vi "Create Repeatability Results Summary Table.vi"(8 "error in (no error)":errorcluster, 11 "Repeatability Results":T1[](array[typedef]) {"Repeatability Percent FS" format="%#_3g"}) -> (0 "error out":errorcluster, 3 "Repeatability Table":string[][](array[string]))   [LabVIEW 2026, in "Analysis.lvlib"]
uses:
  Analysis.lvlib
  Repeatability Result.ctl
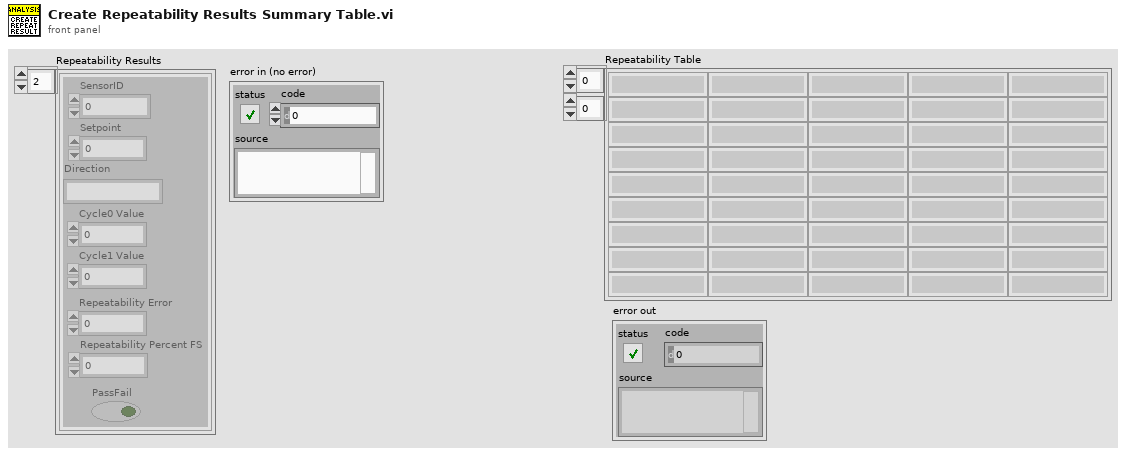
[diagram p1: front panel]
types:
  T1 = typedef "Analysis.lvlib/Repeatability Result.ctl" = cluster{"Setpoint":dbl, "Cycle0 Value":dbl, "SensorID":i32, "Cycle1 Value":dbl, "Repeatability Error":dbl, "Direction":string, "Repeatability Percent FS":dbl, "PassFail":bool}
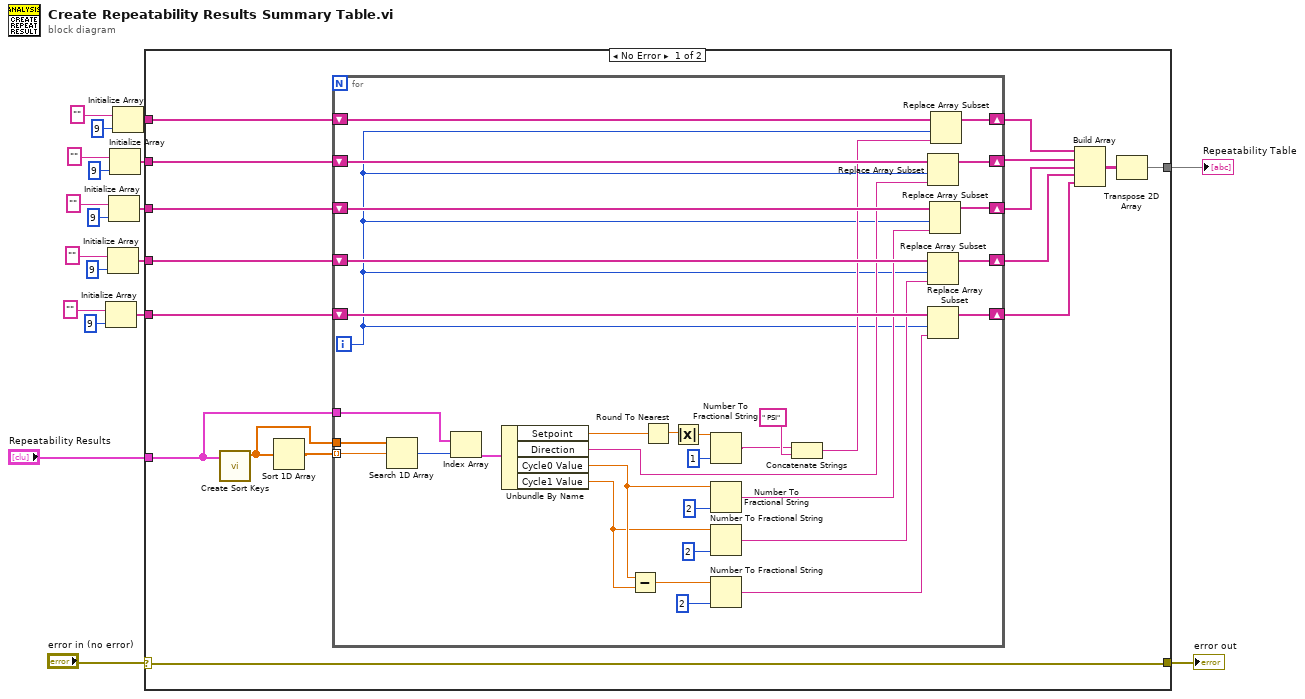
[diagram p0: block diagram]
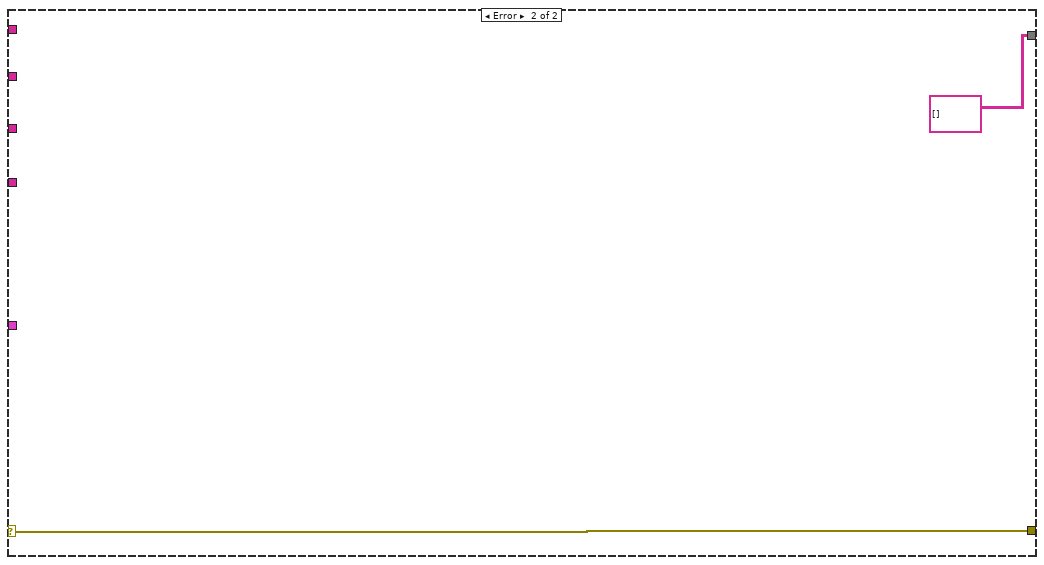
[diagram p2: hidden frame]
diagram:
  n1 = Initialize Array("" ("element"), 9 ("dimension size")) -> (w1:string[])
  n2 = Initialize Array("" ("element"), 9 ("dimension size")) -> (w4:string[])
  n3 = Initialize Array("" ("element"), 9 ("dimension size")) -> (w11:string[])
  n4 = Initialize Array("" ("element"), 9 ("dimension size")) -> (w14:string[])
  n5 = Initialize Array("" ("element"), 9 ("dimension size")) -> (w17:string[])
  n6 = case shown="No Error" "error in (no error)" {
    selector: "error in (no error)" -> [w27 w70]
    tunnel: w17 -> [w35 _]
    tunnel: w14 -> [w34 _]
    tunnel: w11 -> [w33 _]
    tunnel: "Repeatability Results" -> [w21 _]
    tunnel: [w28 string[][] []] -> w10
    tunnel: [w27 w70] -> w8
    tunnel: w4 -> [w26 _]
    tunnel: w1 -> [w24 _]
    frame No Error {
      n7 = call "Create Sort Keys.vi"("Repeatability Results"=w21) -> ("Sort Keys"=w20:dbl[])  [unwired: 9 in, 1 out]
      n8 = Sort 1D Array(array=w20) -> (sorted array=w22:dbl[])
      n9 = for {
        shift-right: [w65] -> w32
        shift-left: w35 -> [w68]
        shift-right: [w66] -> w31
        shift-left: w34 -> [w67]
        shift-right: [w63] -> w30
        shift-left: w33 -> [w64]
        shift-right: [w61] -> w25
        shift-left: w26 -> [w62]
        shift-right: [w59] -> w23
        shift-left: w24 -> [w60]
        tunnel: w22 -> [w52] mode=indexing
        tunnel: w20 -> [w51]
        tunnel: w21 -> [w49]
        i -> [w53]
        n10 = Search 1D Array(1D array=w51, element=w52) -> (index of element=w50:i32)  [unwired: 1 in]
        n11 = Index Array(array=w49, index=w50) -> (element=w36:T1)
        n12 = Unbundle By Name(w36) -> ("Setpoint"=w46:dbl, "Direction"=w57:string, "Cycle0 Value"=w40:dbl, "Cycle1 Value"=w39:dbl)
        n13 = Subtract(x=w40, y=w39) -> (x-y=w37:dbl)
        n14 = Round To Nearest(number=w46) -> (nearest integer value=w44:dbl)
        n15 = Absolute Value(x=w44) -> (abs(x)=w43:dbl)
        n16 = Number To Fractional String(number=w43, precision (6)=i16 1) -> (F-format string=w47:string)  [unwired: 2 in]
        n17 = Number To Fractional String(number=w40, precision (6)=i16 2) -> (F-format string=w56:string)  [unwired: 2 in]
        n18 = Number To Fractional String(number=w39, precision (6)=i16 2) -> (F-format string=w55:string)  [unwired: 2 in]
        n19 = Number To Fractional String(number=w37, precision (6)=i16 2) -> (F-format string=w54:string)  [unwired: 2 in]
        n20 = Concatenate Strings(w47, " PSI" ("element")) -> (w58:string)
        n21 = Replace Array Subset(array=w67, new element=w57, index=w53) -> (w66:string[])
        n22 = Replace Array Subset(array=w62, new element=w55, index=w53) -> (w61:string[])
        n23 = Replace Array Subset(array=w60, new element=w54, index=w53) -> (w59:string[])
        n24 = Replace Array Subset(array=w64, new element=w56, index=w53) -> (w63:string[])
        n25 = Replace Array Subset(array=w68, new element=w58, index=w53) -> (w65:string[])
      }
      n26 = Build Array(w32, w31, w30, w25, w23) -> (w29:string[][])
      n27 = Transpose 2D Array(2D array=w29) -> (transposed array=w28:string[][])
    }
    frame Error {
    }
  }
  "Repeatability Table" <- w10
  "error out" <- w8
